vi "Receive Setpoint.vi"(8 "error in (no error)":errorcluster, 9 "Set Temp":dbl, 11 "Cobra RT in":refnum<class "Cobra RT.lvclass">) -> (0 "error out":errorcluster, 3 "Cobra RT out":refnum<class "Cobra RT.lvclass">)   [LabVIEW 2019, in "Cobra RT.lvlib" / "Cobra RT.lvclass"]
uses:
  Cobra RT.lvclass
  Cobra RT.lvclass/Cobra RT.ctl
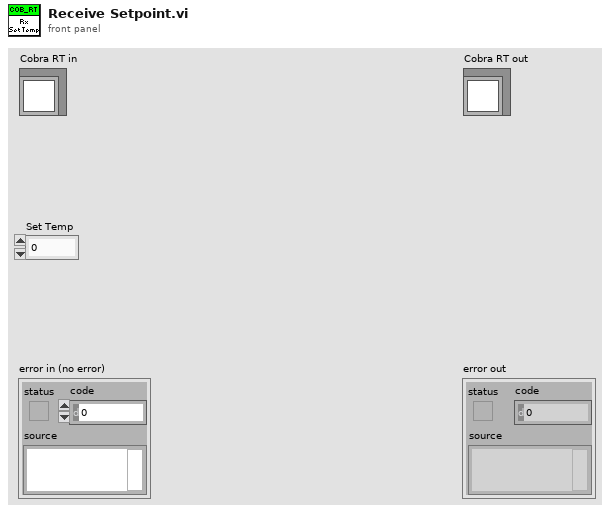
[diagram p1: front panel]
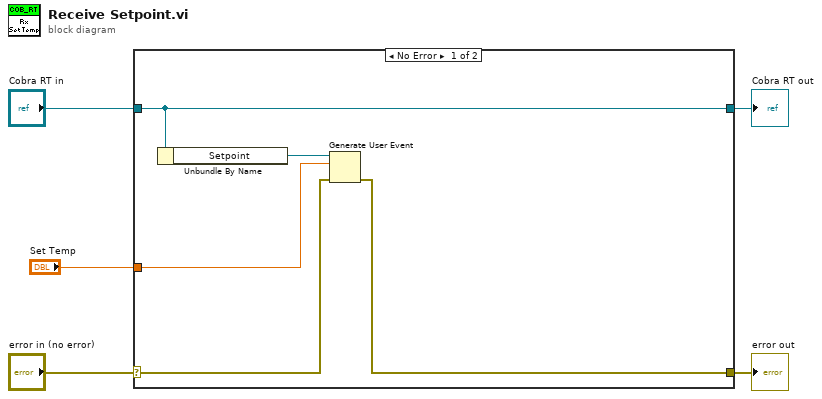
[diagram p0: block diagram]
diagram:
  n1 = case shown="No Error" "error in (no error)" {
    selector: "error in (no error)" -> [w8 w12]
    tunnel: [w7 w12] -> w4
    tunnel: [w10 w11] -> w2
    tunnel: "Cobra RT in" -> [w10 w11]
    tunnel: "Set Temp" -> [w6 _]
    frame No Error {
      n2 = Unbundle By Name(w10) -> ("Setpoint"=w9:refnum<user-event>)
      n3 = Generate User Event(user event=w9, event data cluster=w6, error in=w8) -> (error out=w7:errorcluster)  [unwired: 1 in, 1 out]
    }
    frame Error {
    }
  }
  "error out" <- w4
  "Cobra RT out" <- w2
